vi "AlarmGetState.vi"(11 "Alarm Name":string="Targets/Controller/Alarms/Engine Temperature Alert") -> (0 "error out":errorcluster, 1 "State":T1(ring), 2 "Name":string, 3 "State Text":string)   [LabVIEW 2015, in "ni-veristand-steps-runtime-lib.lvlib"]
uses:
  ni-veristand-steps-runtime-lib.lvlib
  <vilib>/NI Veristand/Execution/Alarm/NI_VS Alarm ExecutionAPI.lvlib
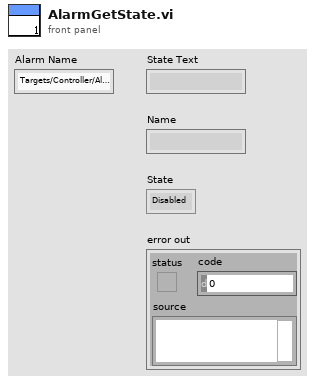
[diagram p1: front panel]
types:
  T1 = enum16{"Disabled", "Enabled", "Tripped", "Delayed Trip", "Indicate"}
  T2 = typedef "NI_VS Alarm ExecutionAPI.lvlib/AlarmAPI.ctl" = refnum<k24>
  T3 = typedef "NI_VS Alarm ExecutionAPI.lvlib/AlarmInfo.ctl" = cluster{"Watch Channel":string, "High Limit Constant":bool, "High Limit Channel":string, "High Limit":dbl, "Low Limit Constant":bool, "Low Limit Channel":string, "Low Limit":dbl, "Procedure Name":string, "Delay":dbl, "Trip Value":dbl, "Priority":enum16{"Low", "Medium", "High"}, "State":enum16{"Disabled", "Enabled", "Tripped", "Delayed Trip", "Indicate"}, "Mode":enum16{"Normal", "Indicate Only"}, "Group Number":u32, "Priority Number":u32, "Name":string, "Full Name":string}
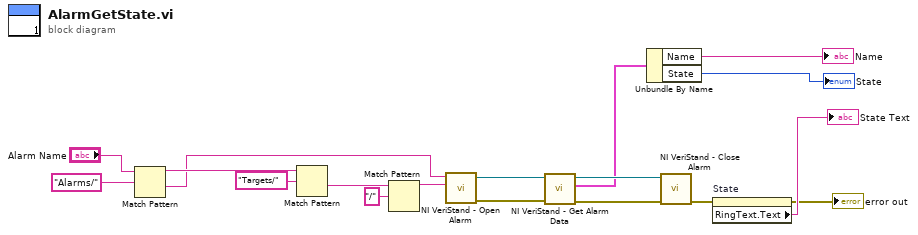
[diagram p0: block diagram]
diagram:
  n1 = Match Pattern(string="Alarm Name", regular expression="Alarms/") -> (before substring=w16:string, after substring=w11:string)  [unwired: 1 in, 2 out]
  n2 = Match Pattern(string=w16, regular expression="Targets/") -> (after substring=w13:string)  [unwired: 1 in, 3 out]
  n3 = Match Pattern(string=w13, regular expression="/") -> (before substring=w12:string)  [unwired: 1 in, 3 out]
  n4 = call <vilib>:"NI VeriStand - Open Alarm.vi"("Target Name (\"\": default target)"=w12, "Alarm Name"=w11) -> ("error out"=w9:errorcluster, "Alarm"=w10:T2)  [unwired: 8 in]
  n5 = call <vilib>:"NI VeriStand - Get Alarm Data.vi"("error in (no error)"=w9, "Alarm in"=w10) -> ("error out"=w8:errorcluster, "Alarm Data"=w6:T3, "Alarm out"=w7:T2)  [unwired: 7 in]
  n6 = Unbundle By Name(w6) -> ("Name"=→"Name":string, "State"=→"State":T1)
  n7 = call <vilib>:"NI VeriStand - Close Alarm.vi"("error in (no error)"=w8, "Alarm"=w7) -> ("error out"=w3:errorcluster)  [unwired: 9 in]
  n8 = property on="State" class="Enum (strict)"(error in=w3) -> (error out=→"error out":errorcluster, "RingText.Text"=→"State Text":string)  [unwired: 1 in, 1 out]
